vi "Lithography Data to Overlay.vi"(8 "error in":errorcluster, 10 "Lithography Data":T2(array[cluster]), 11 "BigMAQ in":refnum<class "BigMAQ.lvclass">) -> (0 "error out":errorcluster, 2 "Disabled Overlays":string[](array[string]), 3 "BigMAQ out":refnum<class "BigMAQ.lvclass">)   [LabVIEW 2019, in "BigMAQ.lvclass"]
uses:
  BigMAQ.lvclass
  <userlib>/LevyLab/Relay Box/Typedefs/Resistor--enum.ctl
  Overlay.ctl
  BigMAQ.lvclass/BigMAQ.ctl
  <userlib>/LevyLab/Relay Box/Relay-Box.lvclass
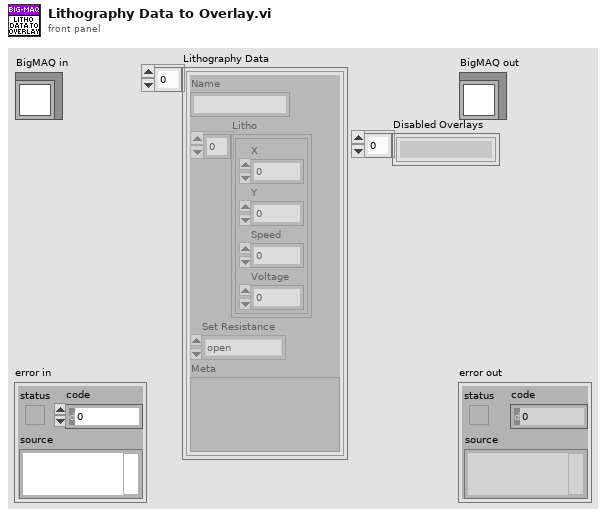
[diagram p1: front panel]
types:
  T1 = typedef "Relay-Box.lvclass/Resistor--enum.ctl" = enum16{"open", "discharge tip", "0 ohms", "100k ohm", "10M ohm", "1G ohm"}
  T2 = cluster{"Name":string, "Litho":cluster{"X":dbl, "Y":dbl, "Speed":dbl, "Voltage":dbl}[], "Set Resistance":T1, "Meta":variant}[]
  T3 = typedef "BigMAQ.lvclass/Overlay.ctl" = cluster{"Name":string, "Data":cluster{"Points":cluster{"X":dbl, "Y":dbl}[], "Voltages":dbl[]}}
  T4 = cluster{"X":dbl, "Y":dbl, "Speed":dbl, "Voltage":dbl}[]
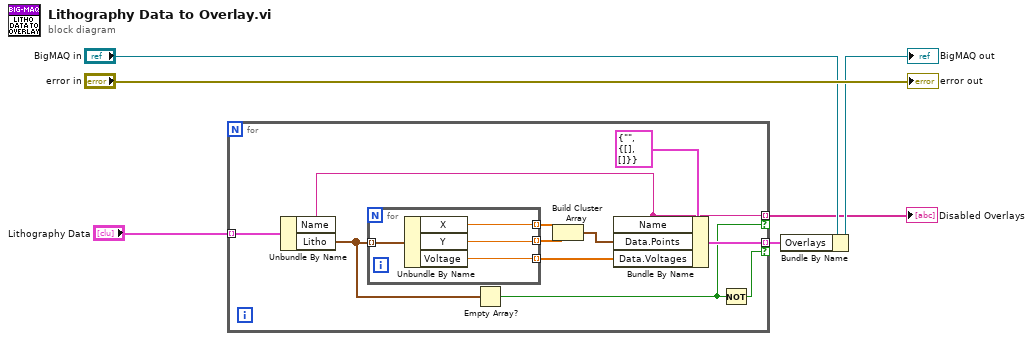
[diagram p0: block diagram]
diagram:
  n1 = for {
    tunnel: "Lithography Data" -> [w17] mode=indexing
    tunnel: [w10] -> w5 mode=indexing if=w7
    tunnel: [w9] -> w1 mode=indexing if=w8
    n2 = Unbundle By Name(w17) -> ("Name"=w9:string, "Litho"=w15:T4)
    n3 = for {
      tunnel: w15 -> [w18] mode=indexing
      tunnel: [w21] -> w14 mode=indexing
      tunnel: [w20] -> w12 mode=indexing
      tunnel: [w19] -> w13 mode=indexing
      n4 = Unbundle By Name(w18) -> ("X"=w20:dbl, "Y"=w19:dbl, "Voltage"=w21:dbl)
    }
    n5 = Empty Array?(array=w15) -> (empty?=w8:bool)
    n6 = Build Cluster Array(w12, w13) -> (w11:cluster{"X":dbl, "Y":dbl}[])
    n7 = Bundle By Name(cluster=T3 {"Name"="", "Data"={"Points"=[], "Voltages"=[]}} ("Overlay"), "Name"=w9, "Data.Points"=w11, "Data.Voltages"=w14) -> (w10:T3)
    n8 = Not(x=w8) -> (.not. x?=w7:bool)
  }
  "Disabled Overlays" <- w1
  n9 = Bundle By Name(cluster="BigMAQ in", "Overlays"=w5) -> (→"BigMAQ out":refnum<class "BigMAQ.lvclass">)
  "error out" <- "error in"
